vi "Configure Frequency Sweep.vi"(0 "VISA resource name":refnum<visa-resource-name>, 1 "Enable Frequency Sweep (T:Enable)":bool, 2 "Sweep Time (1.0 Seconds)":dbl format="%#.6g", 5 "Channel (1: Channel1)":u16(ring) items=["Channel1", "Channel2"], 7 "Sweep Spacing (0: Linear)":u16(ring) items=["Linear", "Logarithmic"], 9 "Start Frequency (1.0 uHz)":dbl format="%#.6g", 11 "error in (no error)":errorcluster, 12 "Stop  Frequency  (1000.0 Hz)":dbl format="%#.6g", 13 "Idle Frequency (0: Start Frequency)":u16(ring) items=["Start Frequency", "Stop Frequency", "DC"]) -> (4 "VISA resource name out":refnum<visa-resource-name>, 15 "error out":errorcluster)   [LabVIEW 2009, in "Agilent 81150.lvlib"]
doc: "Configures and enables a frequency sweep. In the frequency sweep mode, the function generator steps from the start frequency to the stop frequency at a sweep rate."
uses:
  Agilent 81150.lvlib
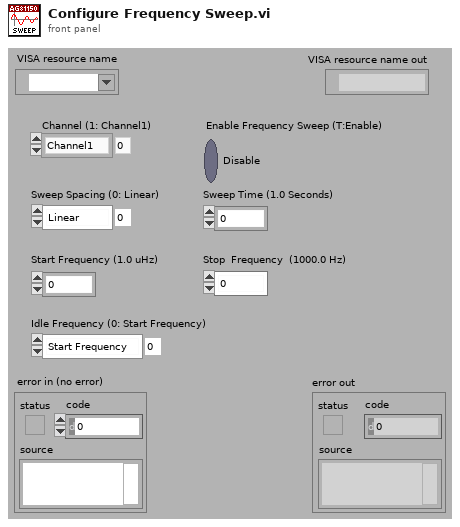
[diagram p1: front panel]
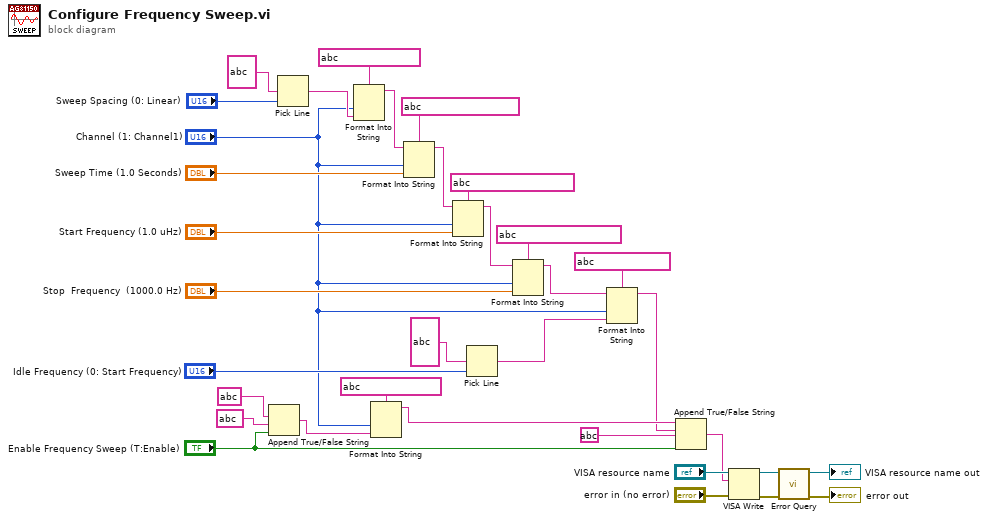
[diagram p0: block diagram]
diagram:
  n1 = Append True/False String(1:"Enable Frequency Sweep (T:Enable)", 2:string ?, 3:string ?) -> (0:w4:string)  [unwired: 1 out]
  n2 = Pick Line(multi-line string=string ?, line index="Sweep Spacing (0: Linear)") -> (output string=w27:string)  [unwired: 1 out]
  n3 = Format Into String(format string=string ?, "Channel (1: Channel1)", w27) -> (resulting string=w20:string)  [unwired: 2 in, 1 out]
  n4 = Format Into String(format string=string ?, "Channel (1: Channel1)", w4) -> (resulting string=w9:string)  [unwired: 2 in, 1 out]
  n5 = Format Into String(format string=string ?, initial string=w20, "Channel (1: Channel1)", "Sweep Time (1.0 Seconds)") -> (resulting string=w14:string)  [unwired: 1 in, 1 out]
  n6 = Format Into String(format string=string ?, initial string=w14, "Channel (1: Channel1)", "Start Frequency (1.0 uHz)") -> (resulting string=w17:string)  [unwired: 1 in, 1 out]
  n7 = Pick Line(multi-line string=string ?, line index="Idle Frequency (0: Start Frequency)") -> (output string=w24:string)  [unwired: 1 out]
  n8 = Format Into String(format string=string ?, initial string=w17, "Channel (1: Channel1)", "Stop  Frequency  (1000.0 Hz)") -> (resulting string=w22:string)  [unwired: 1 in, 1 out]
  n9 = Format Into String(format string=string ?, initial string=w22, "Channel (1: Channel1)", w24) -> (resulting string=w8:string)  [unwired: 1 in, 1 out]
  n10 = Append True/False String(1:"Enable Frequency Sweep (T:Enable)", 2:string ?, 3:w8, 4:w9) -> (0:w7:string)
  n11 = VISA Write(VISA resource name="VISA resource name", write buffer=w7, error in (no error)="error in (no error)") -> (VISA resource name out=w32:refnum<visa-resource-name>, error out=w30:errorcluster)  [unwired: 1 out]
  n12 = call "Error Query.vi"("error in (no error)"=w30, "VISA resource name"=w32) -> ("error out"=→"error out":errorcluster, "VISA resource name out"=→"VISA resource name out":refnum<visa-resource-name>)  [unwired: 8 out]
